vi "SetSampleRate.vi"(8 "error in (no error)":errorcluster, 10 "SampleRate":dbl, 11 "FunctionBase in":refnum<class "FunctionBase.lvclass">) -> (0 "error out":errorcluster, 3 "FunctionBase out":refnum<class "FunctionBase.lvclass">)   [LabVIEW 2018, in "Functions.lvlib" / "FunctionBase.lvclass"]
doc: "IVI Fgen standard does not provide for sample rate contrl, but many of the sub classes need ti so this provides an overridable method to input sample rate."
uses:
  FunctionBase.lvclass
  <userlib>/NIST/BaseClasses/Object_class/BaseObject.lvclass
panel:
  # "IVI Fgen standard does not provide for sample rate contrl, but many of the sub classes need ti so this provides an overridable method to input sample rate."
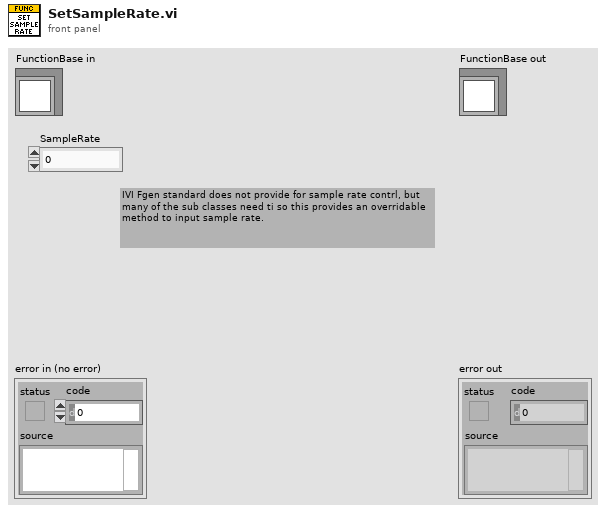
[diagram p1: front panel]
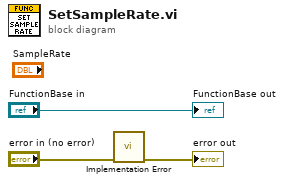
[diagram p0: block diagram]
diagram:
  n1 = call <userlib>:"Implementation Error.vi"("error in (no error)"="error in (no error)") -> ("error out"=→"error out":errorcluster)  [unwired: 10 in]
  "FunctionBase out" <- "FunctionBase in"
